vi "Main.vi"(10 "Sub Panel":refnum<vi>, 11 "Module Admin":refnum<class "Delacor_lib_QMH_Module Admin.lvclass">) -> ()   [LabVIEW 2019, in "Adquisicion_Helper_Loop.lvlib"]
doc: "This template is based off of the Queued Message Handler design pattern and the Queued Message Handler project template that ships with LabVIEW.\n\nThe main difference is that the queue is private to this module and communication between modules is performed via Broadcast and Request events.\n\nRequest events are wrapped in public API methods and are handled in the Event Handling Loop (EHL) of this VI. Any module can register for Broadcast events sent by this module. The EHL generates messages based on user interface actions.\n\nThe Message Handling Loop (MHL) processes messages generated by the EHL, or by other messages. The messages are string values, so new messages can be added easily to the Message Cases case structure in the MHL. Each message cluster can also provide an optional value for Message Data, which is a variant that can be converted to whatever message-specific data is required.\n_____\nBased on Delacor QMH Project Template 5.0.0.82."
uses:
  Adquisicion_Helper_Loop.lvlib
  <vilib>/Delacor/Delacor QMH/Libraries/Module Admin_class/Delacor_lib_QMH_Module Admin.lvclass
  Module Data--cluster.ctl
  Stop helper loop Argument--cluster.ctl
  Stop Argument--cluster.ctl
  <vilib>/Delacor/Delacor QMH/Libraries/Message Queue_class/Delacor_lib_QMH_Message Queue.lvclass/Delacor_lib_QMH_Message Queue.ctl
  <vilib>/Delacor/Delacor QMH/Libraries/Module Admin_class/Delacor_lib_QMH_Module Admin.lvclass/Delacor_lib_QMH_Module Admin.ctl
  <vilib>/Utility/miscctls.llb/LVPointTypeDef.ctl
  <vilib>/Delacor/Delacor QMH/Libraries/Message Queue_class/Delacor_lib_QMH_Enqueue Message (Single).vi
  <vilib>/Delacor/Delacor QMH/Libraries/Module Admin_class/Delacor_lib_QMH_Get External Launch.vi
  <vilib>/Instr/_visa.llb/VISA Configure Serial Port (Instr).vi
  <vilib>/Utility/error.llb/Error Cluster From Error Code.vi
  <vilib>/ErrorRing/Error Ring.xnode
  <vilib>/Delacor/Delacor QMH/Libraries/Message Queue_class/Delacor_lib_QMH_Message Queue.lvclass
  Analisis/Analisis.lvlib
panel:
  out "Aquisition\nBuffer":string
  out "error out":errorcluster
  out "Status":string
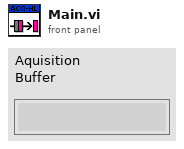
[diagram p1: front panel]
types:
  T1 = typedef "Adquisicion_Helper_Loop.lvlib/Request Events--cluster.ctl" = cluster{"Stop Module":refnum<user-event>, "Show Panel":refnum<user-event>, "Hide Panel":refnum<user-event>, "Get Module Execution Status":refnum<user-event>, "Show Diagram":refnum<user-event>, "Start Helper Loop":refnum<user-event>, "Stop helper loop":refnum<user-event>, "Set Waveform":refnum<user-event>, "Set adquisition parameters":refnum<user-event>}
  T2 = typedef "Adquisicion_Helper_Loop.lvlib/Module Data--cluster.ctl" = cluster{"Status":string}
  T3 = typedef "Adquisicion_Helper_Loop.lvlib/Stop helper loop Argument--cluster.ctl" = cluster{"Boolean":bool}
  T4 = enum32{"invalid lock state", "Not Locked", "Locked (No Password)", "Password-protected"}
  T5 = typedef "Adquisicion_Helper_Loop.lvlib/Stop Argument--cluster.ctl" = cluster{"Origin":string, "Exit via Stop Module Req?":bool, "Wait for Module to stop?":bool}
  T6 = typedef "LVPointTypeDef.ctl" = cluster{"Horizontal":i16, "Vertical":i16}
  T7 = enum32{"Invalid", "Standard", "Closed", "Hidden", "Minimized", "Maximized"}
  T8 = cluster{"Puerto de comunicación":refnum<visa-resource-name>}
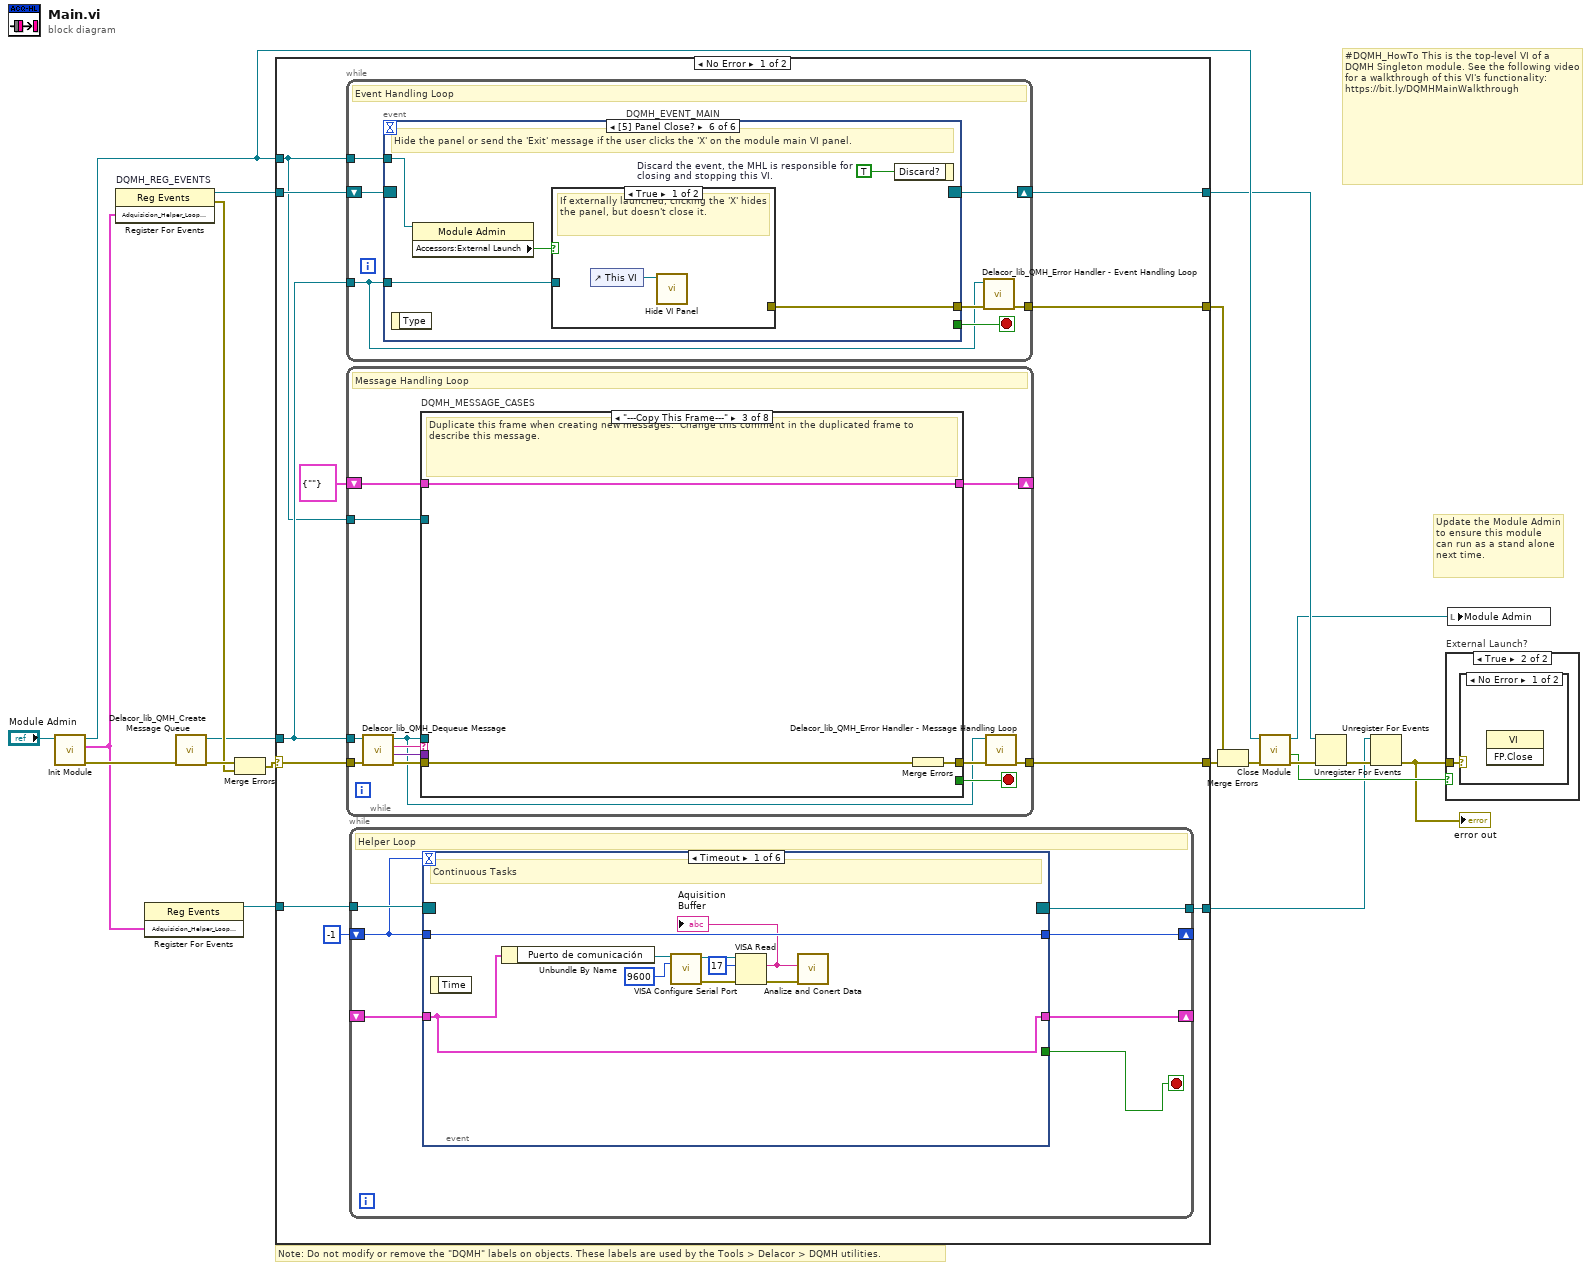
[diagram p0: block diagram]
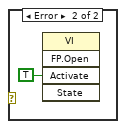
[diagram p3: hidden frame]
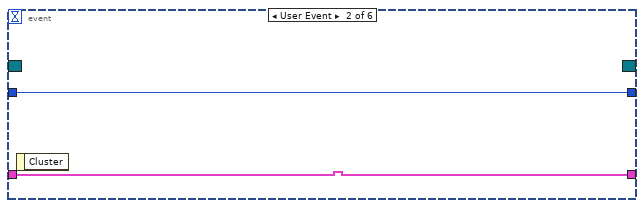
[diagram p4: hidden frame]
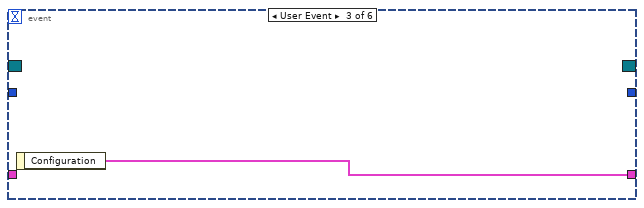
[diagram p5: hidden frame]
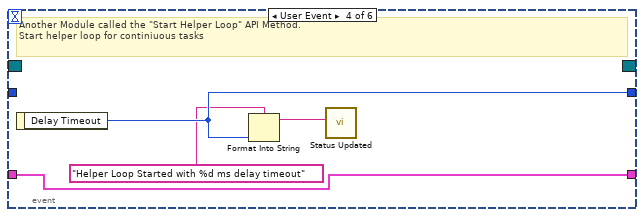
[diagram p6: hidden frame]
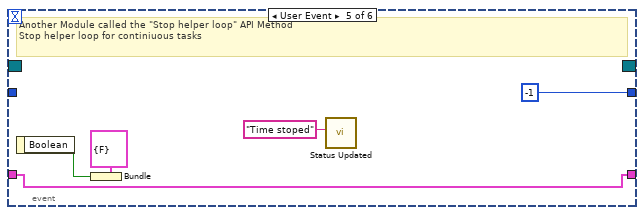
[diagram p7: hidden frame]
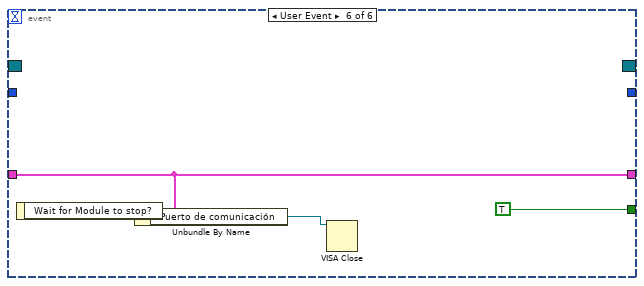
[diagram p8: hidden frame]
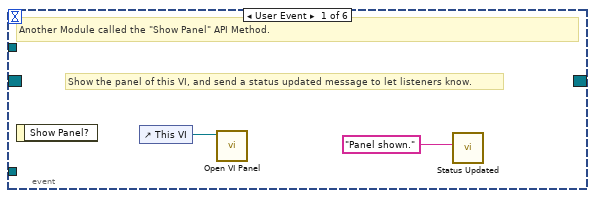
[diagram p9: hidden frame]
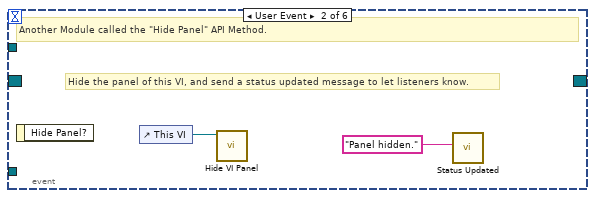
[diagram p10: hidden frame]
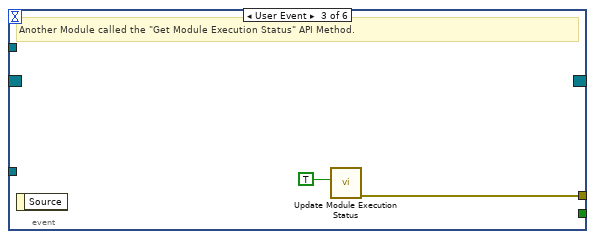
[diagram p11: hidden frame]
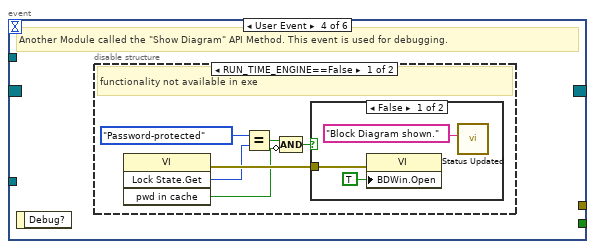
[diagram p12: hidden frame]
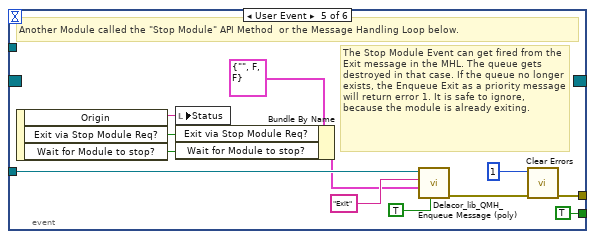
[diagram p15: hidden frame]
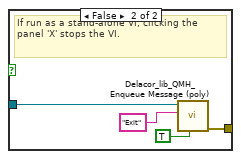
[diagram p16: hidden frame]
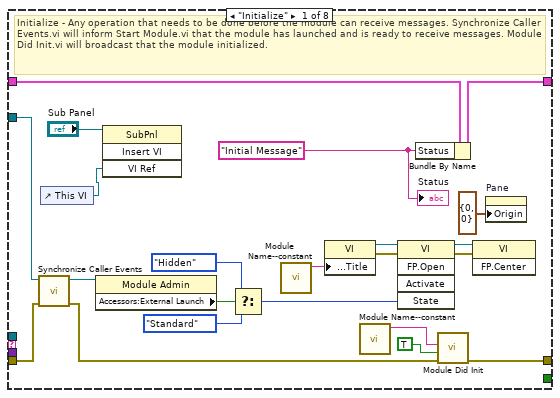
[diagram p17: hidden frame]
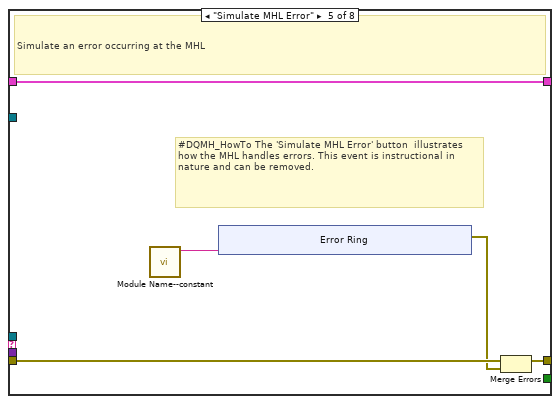
[diagram p20: hidden frame]
diagram:
  # "#DQMH_HowTo This is the top-level VI of a DQMH Singleton module. See the following video for a walkthrough of this VI's functionality: https://bit.ly/DQMHMainWalkthrough"
  # "Note: Do not modify or remove the \"DQMH\" labels on objects. These labels are used by the Tools > Delacor > DQMH utilities."
  # "Update the Module Admin to ensure this module can run as a stand alone next time."
  n1 = call "Init Module.vi"("Singleton Module Admin in"="Module Admin") -> ("error out"=w19:errorcluster, "Adquisicion_Helper_Loop Request Events"=w4:T1, "Singleton Module Admin out"=w12:refnum<class "Delacor_lib_QMH_Module Admin.lvclass">)  [unwired: 8 in]
  n2 = register-events "DQMH_REG_EVENTS"(w4) -> (reference out=w10:refnum<event-registration>, error out=w13:errorcluster)  [unwired: 2 in]
  n3 = register-events(w4) -> (reference out=w5:refnum<event-registration>)  [unwired: 2 in, 1 out]
  n4 = call <vilib>:"Delacor_lib_QMH_Create Message Queue.vi"("error in (no error)"=w19) -> ("error out"=w15:errorcluster, "Message Queue"=w9:refnum<class "Delacor_lib_QMH_Message Queue.lvclass">)  [unwired: 9 in]
  n5 = Merge Errors(w15, w13) -> (w14:errorcluster)
  n6 = case shown="No Error" w14 {
    selector: w14 -> [w29 w208]
    tunnel: [w31 w207] -> w20
    tunnel: [w28 w213] -> w11
    tunnel: w10 -> [w26 w213]
    tunnel: w9 -> [w25 w206]
    tunnel: [w30 _] -> w17
    tunnel: w12 -> [w24 w209]
    tunnel: w5 -> [w23 _]
    tunnel: [w22 _] -> w1
    frame No Error {
      n7 = while {
        tunnel: w25 -> [w63]
        shift-right: [w66] -> w28
        shift-left: w26 -> [w67]
        tunnel: [w68] -> w30
        tunnel: w24 -> [w64]
        stop <- w65 stop-if-true
        # "Event Handling Loop"
        n8 = event "DQMH_EVENT_MAIN" shown="[5] Panel Close?" {
          selector: w67 -> [_ _ _ _ _ _]
          dyn-events: [_ _ _ _ _ _] -> w66
          timeout: _ -> [_ _ _ _ _ _]
          tunnel: [_ _ _ _ TRUE ("Discard?") _] -> w65
          tunnel: w63 -> [_ _ _ _ w92 w99]
          tunnel: [_ _ w75 _ w95 w101] -> w69
          tunnel: w64 -> [_ _ _ _ _ w98]
          event User Event {
            # "Show the panel of this VI, and send a status updated message to let listeners know."
            # "Another Module called the \"Show Panel\" API Method."
            n9 = event-data() -> ()  [unwired: 1 in, 1 out]
            n10 = control-ref of="This VI"() -> (w71:refnum<vi>)
            n11 = call "Open VI Panel.vi"("VI"=w71) -> ()  [unwired: 10 in, 1 out]
            n12 = call "Status Updated.vi"("Status"="Panel shown." ("format string")) -> ()  [unwired: 10 in, 1 out]
          }
          event User Event {
            # "Hide the panel of this VI, and send a status updated message to let listeners know."
            # "Another Module called the \"Hide Panel\" API Method."
            n13 = event-data() -> ()  [unwired: 1 in, 1 out]
            n14 = control-ref of="This VI"() -> (w73:refnum<vi>)
            n15 = call "Hide VI Panel.vi"("VI"=w73) -> ()  [unwired: 10 in, 1 out]
            n16 = call "Status Updated.vi"("Status"="Panel hidden." ("format string")) -> ()  [unwired: 10 in, 1 out]
          }
          event User Event {
            # "Another Module called the \"Get Module Execution Status\" API Method."
            n17 = event-data() -> ()  [unwired: 1 in, 1 out]
            n18 = call "Update Module Execution Status.vi"("Running?"=TRUE) -> ("error out"=w75:errorcluster)  [unwired: 10 in]
          }
          event User Event {
            # "Another Module called the \"Show Diagram\" API Method. This event is used for debugging."
            n19 = event-data() -> ()  [unwired: 1 in, 1 out]
            n20 = disable-structure shown="RUN_TIME_ENGINE==False" {
              frame condition #0 (active) {
                # "functionality not available in exe"
                n21 = invoke class="VI" method="Lock State.Get"() -> (error out=w81:errorcluster, "Get Lock State"=w80:T4, "pwd in cache"=w77:bool)  [unwired: 4 in, 1 out]
                n22 = Equal?(x=T4."Password-protected", y=w80) -> (x = y?=w78:bool)
                n23 = Compound Arithmetic op=AND(w78, invert w77) -> (w76:bool)
                n24 = case shown="False" w76 {
                  tunnel: w81 -> [w84 _]
                  frame False {
                    n25 = property class="VI"(error in=w84, "BDWin.Open"=TRUE ("Block Diagram Window:Open")) -> ()  [unwired: 1 in, 2 out]
                    n26 = call "Status Updated.vi"("Status"="Block Diagram shown." ("format string")) -> ()  [unwired: 10 in, 1 out]
                  }
                  frame True {
                    # "Password-protected VI, and the password is not in the cache. Do not show the diagram."
                  }
                }
              }
              frame condition #1 {
              }
            }
          }
          event User Event {
            # "The Stop Module Event can get fired from the Exit message in the MHL. The queue gets destroyed in that case. If the queue no longer exists, the Enqueue Exit as a priority message will return error 1. It is safe to ignore, because the module is already exiting."
            # "Another Module called the \"Stop Module\" API Method  or the Message Handling Loop below."
            n27 = event-data() -> ("Origin"=w91:string, "Exit via Stop Module Req?"=w87:bool, "Wait for Module to stop?"=w86:bool)  [unwired: 1 in]
            n28 = local write "Status"(w91) -> ()
            n29 = Bundle By Name(cluster=T5 {"Origin"="", "Exit via Stop Module Req?"=FALSE, "Wait for Module to stop?"=FALSE} ("Stop Argument"), "Exit via Stop Module Req?"=w87, "Wait for Module to stop?"=w86) -> (w85:T5)
            n30 = call-poly <vilib>:"Delacor_lib_QMH_Enqueue Message (poly).vi"("Priority Message? (F)"=TRUE, "Message Data"=w85, "Message"="Exit", "Message Queue in"=w92) -> ("error out"=w96:errorcluster)  [unwired: 6 in, 1 out]
            n31 = call <vilib>:"Clear Errors.vi"("error in (no error)"=w96, "specific error code to clear (0: all)"=1) -> ("error out"=w95:errorcluster)  [unwired: 4 in, 1 out]
          }
          event Panel Close? {
            w100 = TRUE  # Discard the event, the MHL is responsible for closing and stopping this VI.
            # "Hide the panel or send the 'Exit' message if the user clicks the 'X' on the module main VI panel."
            n32 = event-data() -> ()  [unwired: 1 in, 1 out]
            n33 = property class="Module Admin"(reference=w98) -> ("Accessors:External Launch"=w97:bool)  [unwired: 1 in, 2 out]
            n34 = case shown="True" w97 {
              tunnel: w99 -> [_ w105]
              tunnel: [_ w106] -> w101
              frame True {
                # "If externally launched, clicking the 'X' hides the panel, but doesn't close it."
                n35 = control-ref of="This VI"() -> (w102:refnum<vi>)
                n36 = call "Hide VI Panel.vi"("VI"=w102) -> ()  [unwired: 10 in, 1 out]
              }
              frame False {
                # "If run as a stand-alone VI, clicking the panel 'X' stops the VI."
                n37 = call-poly <vilib>:"Delacor_lib_QMH_Enqueue Message (poly).vi"("Priority Message? (F)"=TRUE, "Message"="Exit", "Message Queue in"=w105) -> ("error out"=w106:errorcluster)  [unwired: 7 in, 1 out]
              }
            }
            n38 = event-data("Discard?"=w100) -> ()  [unwired: 1 in, 1 out]
          }
        }
        n39 = call-dynamic "Delacor_lib_QMH_Error Handler - Event Handling Loop.vi"("error in (no error)"=w69, "Message Queue in"=w63) -> ("dup error in"=w68:errorcluster)  [unwired: 8 in, 1 out]
      }
      n40 = while {
        tunnel: w25 -> [w109]
        shift-right: [w113] -> _
        shift-left: T2 {"Status"=""} ("Data Cluster") -> [w114]
        tunnel: w29 -> [w117]
        tunnel: [w115] -> w31
        tunnel: w24 -> [w107]
        stop <- w112 stop-if-true
        # "Message Handling Loop"
        n41 = call-dynamic "Delacor_lib_QMH_Dequeue Message.vi"("error in (no error)"=w117, "Message Queue in"=w109) -> ("error out"=w116:errorcluster, "Message Data"=w110:variant, "Message"=w111:string, "Message Queue out"=w108:refnum<class "Delacor_lib_QMH_Message Queue.lvclass">)  [unwired: 6 in]
        n42 = case "DQMH_MESSAGE_CASES" shown="\"---Copy This Frame---\"" w111 {
          selector: w111 -> [_ _ _ _ _ _ _ w193]
          tunnel: w108 -> [_ _ _ _ _ w163 w185 _]
          tunnel: w116 -> [w138 w142 w145 w147 w152 w170 w191 w195]
          tunnel: [w136 w142 w144 w147 w151 w166 w188 w196] -> w118
          tunnel: w114 -> [w127 w141 w143 w146 w149 w165 w184 w194]
          tunnel: [w126 w141 w143 w146 w149 w165 w184 w194] -> w113
          tunnel: [_ _ _ _ _ _ w183 _] -> w112
          tunnel: w110 -> [_ _ _ _ _ w164 w182 _]
          tunnel: w107 -> [w128 _ _ _ _ w162 w177 _]
          frame "Initialize" {
            w121 = "Initial Message" ("Initial Message")
            # "Initialize - Any operation that needs to be done before the module can receive messages. Synchronize Caller Events.vi will inform Start Module.vi that the module has launched and is ready to receive messages. Module Did Init.vi will broadcast that the module initialized."
            n43 = call "Synchronize Caller Events.vi"("error in (no error)"=w138, "Singleton Module Admin in"=w128) -> ("error out"=w137:errorcluster, "Singleton Module Admin out"=w123:refnum<class "Delacor_lib_QMH_Module Admin.lvclass">)  [unwired: 8 in]
            n44 = control-ref of="This VI"() -> (w119:refnum<vi>)
            n45 = property class="Module Admin"(reference=w123) -> ("Accessors:External Launch"=w132:bool)  [unwired: 1 in, 2 out]
            n46 = invoke class="SubPnl" method="Insert VI"(reference="Sub Panel", "VI Ref"=w119) -> ()  [unwired: 2 in, 4 out]
            n47 = Select(t=T7."Hidden" ("State"), s=w132, f=T7."Standard" ("State")) -> (s? t:f=w129:T7)
            n48 = call "Module Name--constant.vi"() -> ("Module Name"=w135:string)  [unwired: 11 in]
            n49 = property class="VI"("Front Panel.Title"=w135) -> (reference out=w134:refnum<vi>, error out=w140:errorcluster)  [unwired: 2 in]
            n50 = call "Module Name--constant.vi"() -> ("Module Name"=w124:string)  [unwired: 11 in]
            n51 = invoke class="VI" method="FP.Open"(reference=w134, error in=w140, "State"=w129) -> (reference out=w133:refnum<vi>, error out=w139:errorcluster)  [unwired: 2 in, 3 out]
            n52 = Bundle By Name(cluster=w127, "Status"=w121) -> (w126:T2)
            n53 = call "Module Did Init.vi"("error in (no error)"=w137, "Initialized?"=TRUE, "Origin"=w124) -> ("error out"=w136:errorcluster)  [unwired: 8 in]
            n54 = invoke class="VI" method="FP.Center"(reference=w133, error in=w139) -> ()  [unwired: 1 in, 3 out]
            n55 = property on="Pane" class="Pane"("Origin"=T6 {"Horizontal"=0, "Vertical"=0}) -> ()  [unwired: 2 in, 2 out]
            "Status" <- w121
          }
          frame "--- Module Specific ---" {
            # "Separator -- The following cases handle messages specific to this Module."
          }
          frame "---Copy This Frame---" {
            # "Duplicate this frame when creating new messages.  Change this comment in the duplicated frame to describe this message."
            n56 = Merge Errors(w145) -> (w144:errorcluster)
          }
          frame "--- Exit and Error Handling---" {
            # "Separator - The following cases handle errors and exit messages."
          }
          frame "Simulate MHL Error" {
            # "#DQMH_HowTo The 'Simulate MHL Error' button  illustrates how the MHL handles errors. This event is instructional in nature and can be removed."
            # "Simulate an error occurring at the MHL"
            n57 = call "Module Name--constant.vi"() -> ("Module Name"=w148:string)  [unwired: 11 in]
            n58 = xnode "Error Ring"("parameter 0"=w148) -> ("error out"=w150:errorcluster)
            n59 = Merge Errors(w152, w150) -> (w151:errorcluster)
          }
          frame "Error" {
            # "#CodeRecommended - If you ever change the name of this \"Error\" message, you'll need to update the name in the Check Loop Error.vi as well."
            # "#CodeRecommended - If the module is running in standalone mode (External Launch = FALSE), this code will pop up an error dialog and call the 'Exit' message if an error occurs. Add more fine-grained error handling here."
            # "Error - Check the error message data and respond accordingly. This message is sent by the \"Error Handler\" VIs at the end of each loop in this application."
            n60 = property class="Module Admin"(reference=w162) -> ("Accessors:External Launch"=w161:bool)  [unwired: 1 in, 2 out]
            n61 = Variant To Data(error in=w170, type=errorcluster {"status"=FALSE, "code"=0, "source"=""} ("error constant"), Variant=w164) -> (data=w171:errorcluster, error out=w168:errorcluster)
            n62 = call "Module Name--constant.vi"() -> ("Module Name"=w160:string)  [unwired: 11 in]
            n63 = call "Error Reported.vi"("Additional Information"=w160, "Error"=w171) -> ()  [unwired: 9 in, 1 out]
            n64 = case shown="False" w161 {
              tunnel: [w176 _] -> w167
              tunnel: w163 -> [w174 _]
              tunnel: w171 -> [w175 _]
              frame False {
                # "If the module is running standalone, then pop up an error dialog and call the \"Exit\" message."
                n65 = call <vilib>:"Simple Error Handler.vi"("error in (no error)"=w175) -> ()  [unwired: 4 in, 5 out]
                n66 = call-poly <vilib>:"Delacor_lib_QMH_Enqueue Message (poly).vi"("Priority Message? (F)"=TRUE, "Message"="Exit", "Message Queue in"=w174) -> ("error out"=w176:errorcluster)  [unwired: 7 in, 1 out]
              }
              frame True {
                # "If the module was launched externally, calling the Error Reported broadcast VI is the only action performed by the \"Error\" message. The module's caller can then process the error appropriately."
              }
            }
            n67 = Merge Errors(w168, w167) -> (w166:errorcluster)
            n68 = local write "error out"(w166) -> ()
          }
          frame "Exit" {
            w181 = 91  # 91: not all Exit messages will have an argument
            w183 = TRUE  # Stop the VI
            # "Release the message queue reference"
            # "#CodeNeeded - Add any required cleanup code here"
            # "Exit - Exit the application."
            n69 = Variant To Data(error in=w191, type=T5 {"Origin"="", "Exit via Stop Module Req?"=FALSE, "Wait for Module to stop?"=FALSE} ("Stop Argument"), Variant=w182) -> (data=w179:T5, error out=w187:errorcluster)
            n70 = call <vilib>:"Clear Errors.vi"("error in (no error)"=w187, "specific error code to clear (0: all)"=w181) -> ("error out"=w190:errorcluster)  [unwired: 4 in, 1 out]
            n71 = control-ref of="This VI"() -> (w178:refnum<vi>)
            n72 = call-dynamic "Delacor_lib_QMH_Release Message Queue.vi"("error in (no error)"=w190, "Message Queue"=w185) -> ("error out"=w189:errorcluster)  [unwired: 9 in]
            n73 = call "Handle Exit.vi"("Stop Argument"=w179, "Admin in"=w177, "VI reference"=w178) -> ("error out"=w186:errorcluster)  [unwired: 7 in, 1 out]
            n74 = Merge Errors(w189, w186) -> (w188:errorcluster)
          }
          frame Default {
            # "'Default' case only runs if there is a message that isn't defined in any of the other cases.  Output a programming error."
            n75 = call "Module Name--constant.vi"() -> ("Module Name"=w192:string)  [unwired: 11 in]
            n76 = xnode "Error Ring"("parameter 0"=w193, "parameter 1"=w192) -> ("error out"=w197:errorcluster)
            n77 = Merge Errors(w195, w197) -> (w196:errorcluster)
          }
        }
        n78 = call-dynamic "Delacor_lib_QMH_Error Handler - Message Handling Loop.vi"("error in (no error)"=w118, "Message Queue in"=w108) -> ("dup error in"=w115:errorcluster)  [unwired: 8 in, 1 out]
      }
      n79 = while {
        tunnel: w23 -> [w38]
        tunnel: [w37] -> w22
        shift-right: [w36] -> _
        shift-left: -1 -> [w35]
        shift-right: [w33] -> _
        shift-left: _ -> [w32]
        stop <- w34 stop-if-true
        # "Helper Loop"
        n80 = event shown="[0] Timeout" {
          selector: w38 -> [_ _ _ _ _ _]
          dyn-events: [_ _ _ _ _ _] -> w37
          timeout: w35 -> [_ _ _ _ _ _]
          tunnel: [w47 w49 _ w54 -1 _] -> w36
          tunnel: w35 -> [w47 w49 _ _ _ _]
          tunnel: [_ _ _ _ _ TRUE] -> w34
          tunnel: [w41 w48 w50 w51 w55 w61] -> w33
          tunnel: w32 -> [w41 w48 _ w51 w55 w61]
          event Timeout {
            # "Continuous Tasks"
            n81 = event-data() -> ()  [unwired: 1 in, 1 out]
            n82 = Unbundle By Name(w41) -> ("Puerto de comunicación"=w46:refnum<visa-resource-name>)
            n83 = call-poly "VISA Configure Serial Port"("VISA resource name"=w46, "baud rate (9600)"=u32 9600) -> ("VISA resource name out"=w45:refnum<visa-resource-name>, "error out"=w44:errorcluster)  [unwired: 12 in]
            n84 = VISA Read(VISA resource name=w45, byte count=u32 17, error in (no error)=w44) -> (read buffer=w40:string, error out=w39:errorcluster)  [unwired: 2 out]
            "Aquisition\nBuffer" <- w40
            n85 = call "Analize and Conert Data.vi"("error in (no error)"=w39, "Data"=w40) -> ()  [unwired: 9 in, 1 out]
          }
          event User Event {
            n86 = event-data() -> ()  [unwired: 1 in, 1 out]
          }
          event User Event {
            n87 = event-data() -> ("Configuration"=w50:T8)  [unwired: 1 in]
          }
          event User Event {
            # "Another Module called the \"Start Helper Loop\" API Method.\nStart helper loop for continiuous tasks"
            n88 = event-data() -> ("Delay Timeout"=w54:i32)  [unwired: 1 in]
            n89 = Format Into String(format string="Helper Loop Started with %d ms delay timeout", w54) -> (resulting string=w52:string)  [unwired: 2 in, 1 out]
            n90 = call "Status Updated.vi"("Status"=w52) -> ()  [unwired: 10 in, 1 out]
          }
          event User Event {
            # "Another Module called the \"Stop helper loop\" API Method\nStop helper loop for continiuous tasks"
            n91 = event-data() -> ("Boolean"=w58:bool)  [unwired: 1 in]
            n92 = Bundle(cluster=T3 {"Boolean"=FALSE} ("Stop helper loop Argument"), "Boolean"=w58) -> ()  [unwired: 1 out]
            n93 = call "Status Updated.vi"("Status"="Time stoped") -> ()  [unwired: 10 in, 1 out]
          }
          event User Event {
            n94 = event-data() -> ()  [unwired: 1 in, 1 out]
            n95 = Unbundle By Name(w61) -> ("Puerto de comunicación"=w60:refnum<visa-resource-name>)
            n96 = VISA Close(VISA resource name=w60) -> ()  [unwired: 1 in, 1 out]
          }
        }
      }
    }
    frame Error {
      # "Synchronize Caller Events.vi will inform Start Module.vi that the module has launched and will let the code calling Start Module.vi register for broadcasts and would permit the caller receive the broadcast that an error occurred at launch time."
      n97 = call-dynamic "Delacor_lib_QMH_Release Message Queue.vi"("error in (no error)"=w208, "Message Queue"=w206) -> ("error out"=w207:errorcluster)  [unwired: 9 in]
      n98 = call "Synchronize Caller Events.vi"("Singleton Module Admin in"=w209) -> ("error out"=w214:errorcluster)  [unwired: 9 in, 1 out]
      n99 = call "Module Name--constant.vi"() -> ("Module Name"=w212:string)  [unwired: 11 in]
      n100 = Format Into String(format string="An error occurred during initialization. %s is no longer running.", w212) -> (resulting string=w210:string)  [unwired: 2 in, 1 out]
      n101 = Merge Errors(w207, w214) -> (w215:errorcluster)
      n102 = call "Error Reported.vi"("Additional Information"=w210, "Error"=w215) -> ()  [unwired: 9 in, 1 out]
    }
  }
  n103 = Merge Errors(w17, w20) -> (w16:errorcluster)
  n104 = call "Close Module.vi"("error in (no error)"=w16, "Module Admin in"=w12) -> ("error out"=w18:errorcluster, "External Launch"=w6:bool, "Module Admin out"=w7:refnum<class "Delacor_lib_QMH_Module Admin.lvclass">)  [unwired: 7 in]
  n105 = Unregister For Events(event registration refnum=w11, error in=w18) -> (error out=w3:errorcluster)
  n106 = Unregister For Events(event registration refnum=w1, error in=w3) -> (error out=w2:errorcluster)
  "error out" <- w2
  n107 = case "External Launch?" shown="True" w6 {
    tunnel: w2 -> [_ w216]
    frame False {
    }
    frame True {
      n108 = case shown="No Error" w216 {
        frame No Error {
          n109 = invoke class="VI" method="FP.Close"() -> ()  [unwired: 3 in, 3 out]
        }
        frame Error {
          n110 = invoke class="VI" method="FP.Open"("Activate"=TRUE ("Activate?")) -> ()  [unwired: 4 in, 5 out]
        }
      }
    }
  }
  n111 = local write "Module Admin"(w7) -> ()
